vi "Pneumatic Press and Hold.vi"   [LabVIEW 2013]
uses:
  <vilib>/Rock Robotics/WPI/Solenoid/WPI_SolenoidOpenSingle.vi
  <vilib>/Rock Robotics/WPI/Solenoid/WPI_SolenoidSetEnum.vi
  <vilib>/Rock Robotics/WPI/Solenoid/WPI_SolenoidValue.ctl
  Sally_Framework_2014/Robot Global Data.vi
types:
  T1 = typedef "WPI_SolenoidDevRef.ctl" = cluster{"DevStatus":errorcluster, "Solenoid Module":T2, "Forward Solenoid Channel":T3, "Reverse Solenoid Channel":T3}
  T2 = typedef "FPGA_TypedefSolenoidModule.ctl" = enum16{"Solenoid Module 1", "Solenoid Module 2"}
  T3 = typedef "WPI_SolenoidChannel.ctl" = enum8{"Solenoid 1", "Solenoid 2", "Solenoid 3", "Solenoid 4", "Solenoid 5", "Solenoid 6", "Solenoid 7", "Solenoid 8", "Invalid"}
  T4 = typedef "WPI_SolenoidValue.ctl" = enum16{"Off", "On", "Forward", "Reverse"}
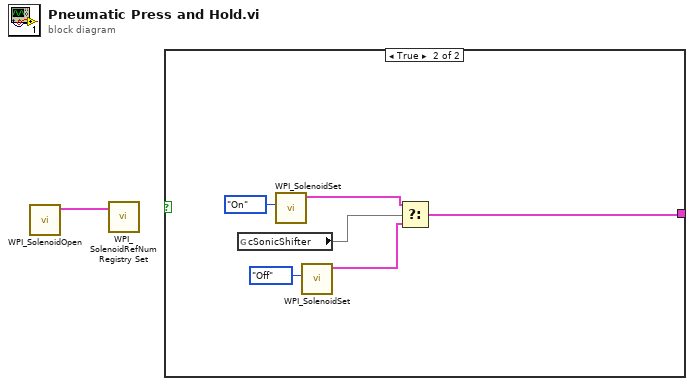
[diagram p0: block diagram]
diagram:
  n1 = call-poly <vilib>:"WPI_SolenoidOpen.vi"() -> ("SolenoidDevRef"=w1:T1)  [unwired: 10 in, 1 out]
  n2 = call <vilib>:"WPI_SolenoidRefNum Registry Set.vi"("SolenoidDevRef"=w1) -> ()  [unwired: 9 in, 2 out]
  n3 = case shown="True" {
    selector: _ -> [_ _]
    tunnel: [_ w2] -> _
    frame False {
    }
    frame True {
      n4 = global read "Robot Global Data.vi" "cSonicShifter"() -> (w3)
      n5 = call-poly <vilib>:"WPI_SolenoidSet.vi"("Value"=WPI_SolenoidValue."On") -> ("SolenoidDevRef"=w6:T1)  [unwired: 9 in, 1 out]
      n6 = call-poly <vilib>:"WPI_SolenoidSet.vi"("Value"=WPI_SolenoidValue."Off") -> ("SolenoidDevRef"=w4:T1)  [unwired: 9 in, 1 out]
      n7 = Select(t=w6, s=w3, f=w4) -> (s? t:f=w2:T1)
    }
  }
